vi "matlab_TI2_moveUpdate.vi"(8 "error in (no error)":errorcluster, 10 "Position counter":i32, 11 "Saved positions":dbl[][](array[numeric])) -> (0 "error out":errorcluster, 2 "XYZpos":cluster{dbl, dbl, dbl})   [LabVIEW 2018]
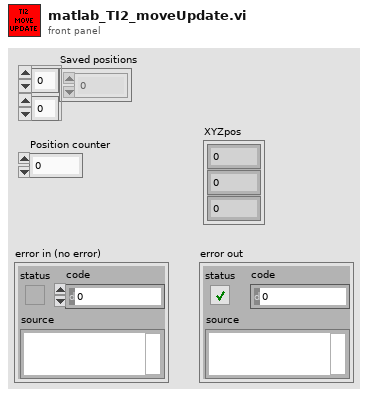
[diagram p1: front panel]
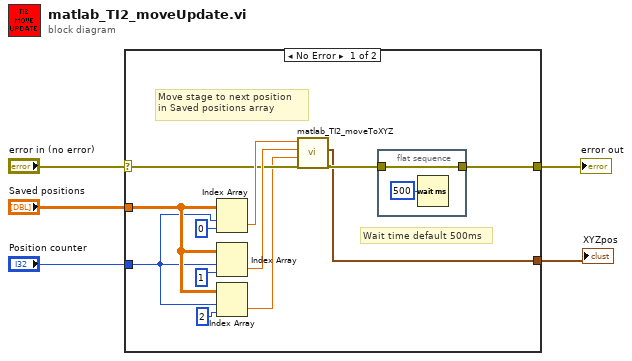
[diagram p0: block diagram]
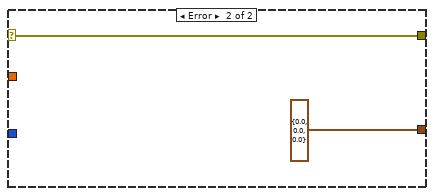
[diagram p2: hidden frame]
diagram:
  n1 = case shown="No Error" "error in (no error)" {
    selector: "error in (no error)" -> [w13 w21]
    tunnel: [w17 w21] -> w5
    tunnel: "Position counter" -> [w7 _]
    tunnel: "Saved positions" -> [w8 _]
    tunnel: [w11 cluster{dbl, dbl, dbl} {0.0, 0.0, 0.0} ("XYZpos")] -> w1
    frame No Error {
      # "Wait time default 500ms"
      # "Move stage to next position \nin Saved positions array"
      n2 = Index Array(array=w8, index (row)=w7, index (col)=0 ("disabled index (col)")) -> (element=w14:dbl)
      n3 = Index Array(array=w8, index (row)=w7, index (col)=1 ("disabled index (col)")) -> (element=w15:dbl)
      n4 = Index Array(array=w8, index (row)=w7, index (col)=2 ("disabled index (col)")) -> (element=w6:dbl)
      n5 = call "matlab_TI2_moveToXYZ.vi"("error in"=w13, "zset"=w6, "yset"=w15, "xset"=w14) -> ("error out"=w12:errorcluster, "XYZpos"=w11:cluster{dbl, dbl, dbl})  [unwired: 6 in]
      n6 = flat-sequence {
        tunnel: w12 -> [w18]
        tunnel: [w18] -> w17
        frame #0 {
          n7 = Wait (ms)(milliseconds to wait=u32 500) -> ()  [unwired: 1 out]
        }
      }
    }
    frame Error {
    }
  }
  "error out" <- w5
  "XYZpos" <- w1
